vi "Unpack for gRPC.vi"(8 "error in":errorcluster, 9 "configuration / results":enum16{"Configuration", "Results"}(ring), 10 "any":T1, 11 "measurement customizations in":refnum<class "Measurement Plugin.lvclass">) -> (0 "error out":errorcluster, 2 "data value":variant, 3 "measurement customizations out":refnum<class "Measurement Plugin.lvclass">)   [LabVIEW 2021, in "Line Transient Response with Pin Map.lvlib" / "Measurement Plugin.lvclass"]
uses:
  Measurement Plugin.lvclass
  Measurement Configuration.ctl
  Line Transient Response with Pin Map.lvlib
  Measurement Results.ctl
  3ecd018e-d556-4cbc-bc60-c4ba57204520.vi
  a521b266-ce99-437c-923d-067dcf1e07fd.vi
  <vilib>/Plug-In SDKs/Measurements/Measurement Plugin Service/Measurement Plugin Service.lvclass
  <instrlib>/niScope/Controls/niScope vertical coupling.ctl
  <vilib>/gRPC/LabVIEW gRPC Library/Shared/Any.ctl
  <vilib>/gRPC/LabVIEW gRPC Library/grpc-lvsupport-release.lvlib
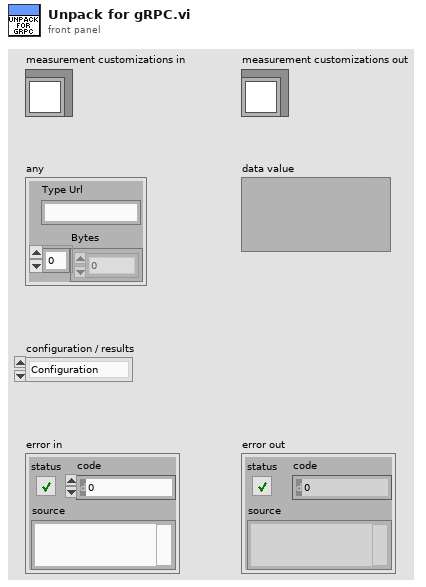
[diagram p1: front panel]
types:
  T1 = typedef "grpc-lvsupport-release.lvlib/Any.ctl" = cluster{"Type Url":string, "Bytes":u8[]}
  T2 = typedef "grpc-lvsupport-release.lvlib/grpcId.ctl" = u64
  T3 = typedef "Line Transient Response with Pin Map.lvlib/Measurement Configuration.ctl" = cluster{"DUT setup time":dbl, "Nominal output voltage":dbl, "Source pin name":string, "Source current limit":dbl, "Source maximum power":dbl, "Source sample rate":dbl, "Source voltage set point 1":dbl, "Source voltage set point 2":dbl, "Source voltatge pulse duration":dbl, "Source voltage delay t1":dbl, "Source voltage delay t2":dbl, "Source voltage falling slew rate":dbl, "Source voltage rising slew rate":dbl, "Source transient response":i32, "Source voltage gain bandwidth":dbl, "Source voltage compensation frequency":dbl, "Source voltage pole-zero ratio":dbl, "Load pin name":string, "Load voltage limit range":dbl, "Load current level range":dbl, "Load current level":dbl, "Load transient response":i32, "Load current gain bandwidth":dbl, "Load current compensation frequency":dbl, "Load current pole-zero ratio":dbl, "Pin Names for Scope":string[], "vertical range":dbl[], "vertical offset":dbl[], "probe attenuation":dbl[], "vertical coupling":T4[], "channel enabled":bool[], "input impedance":u32[], "max input frequency":dbl[], "min sample rate":dbl[], "reference position":dbl[], "min record length":i32[], "enforce realtime":bool[]}
  T4 = typedef "niScope vertical coupling.ctl" = i32
  T5 = typedef "Line Transient Response with Pin Map.lvlib/Measurement Results.ctl" = cluster{"dt":dbl, "Load voltages":dbl[], "Undershoot load voltage":dbl, "Overshoot load voltage":dbl, "Source voltages":dbl[], "waveform pins":string[], "waveform sites":i32[], "waveform t0 array":dbl[], "waveform dt array":dbl[], "waveform length array":i32[], "concatenated waveform Y":dbl[]}
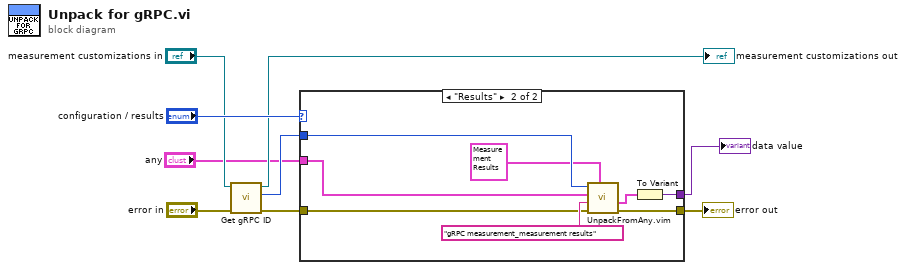
[diagram p0: block diagram]
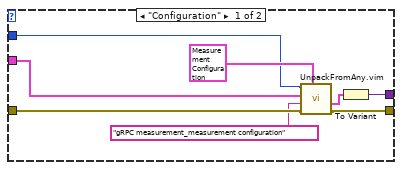
[diagram p2: hidden frame]
diagram:
  n1 = call <vilib>:"Get gRPC ID.vi"("error in"="error in", "measurement plugin service in"="measurement customizations in") -> ("error out"=w6:errorcluster, "gRPC ID"=w3:T2, "measurement plugin service out"=→"measurement customizations out":refnum<class "Measurement Plugin.lvclass">)  [unwired: 7 in]
  n2 = case shown="\"Results\"" "configuration / results" {
    tunnel: w6 -> [w15 w19]
    tunnel: "any" -> [w10 w18]
    tunnel: w3 -> [w12 w22]
    tunnel: [w16 w23] -> w9
    tunnel: [w17 w25] -> w1
    frame "Configuration" {
      n3 = call "UnpackFromAny.vim"("Data Type"=T3 {"DUT setup time"=32.0, "Nominal output voltage"=1.0, "Source pin name"="Lorem ipsum dolor sit", "Source current limit"=1.2, "Source maximum power"=6.0, "Source sample rate"=1.0, "Source voltage set point 1"=20.0, "Source voltage set point 2"=20.0, "Source voltatge pulse duration"=0.005, "Source voltage delay t1"=0.005, "Source voltage delay t2"=0.005, "Source voltage falling slew rate"=-32.0, "Source voltage rising slew rate"=24.0, "Source transient response"=1042, "Source voltage gain bandwidth"=2000.0, "Source voltage compensation frequency"=3530.0, "Source voltage pole-zero ratio"=2.0, "Load pin name"="", "Load voltage limit range"=6.0, "Load current level range"=1.0, "Load current level"=1.0, "Load transient response"=1042, "Load current gain bandwidth"=14000.0, "Load current compensation frequency"=180000.0, "Load current pole-zero ratio"=0.3, "Pin Names for Scope"=[], "vertical range"=[], "vertical offset"=[], "probe attenuation"=[], "vertical coupling"=[], "channel enabled"=[], "input impedance"=[], "max input frequency"=[], "min sample rate"=[], "reference position"=[], "min record length"=[], "enforce realtime"=[]} ("Measurement Configuration"), "error in"=w15, "Message Type"="gRPC measurement_measurement configuration", "Any"=w10, "gRPCid in"=w12) -> ("error out"=w16:errorcluster, "Unpacked Value"=w14:T3)  [unwired: 4 in, 1 out]
      n4 = To Variant(anything=w14) -> (Variant=w17:variant)
    }
    frame "Results" {
      n5 = call "UnpackFromAny.vim"("Data Type"=T5 {"dt"=0.0, "Load voltages"=[], "Undershoot load voltage"=0.0, "Overshoot load voltage"=0.0, "Source voltages"=[0.0], "waveform pins"=[], "waveform sites"=[], "waveform t0 array"=[], "waveform dt array"=[], "waveform length array"=[], "concatenated waveform Y"=[]} ("Measurement Results"), "error in"=w19, "Message Type"="gRPC measurement_measurement results", "Any"=w18, "gRPCid in"=w22) -> ("error out"=w23:errorcluster, "Unpacked Value"=w24:T5)  [unwired: 4 in, 1 out]
      n6 = To Variant(anything=w24) -> (Variant=w25:variant)
    }
  }
  "error out" <- w9
  "data value" <- w1
